vi "ep_Check Signaling Freuquency.vi"(8 "error in (no error)":errorcluster, 9 "nominal frequency value":dbl, 10 "phase voltage spectra":T2(array[cluster]), 11 "signaling frequency [Hz]":dbl) -> (0 "error out":errorcluster)   [LabVIEW 2014, in "NI_EP_Power Quality.lvlib"]
uses:
  <vilib>/addons/Electrical Power/PQ/NI_EP_Power Quality.lvlib
  <vilib>/addons/Electrical Power/PQ/Common/Controls/ep_AI Data Channel.ctl
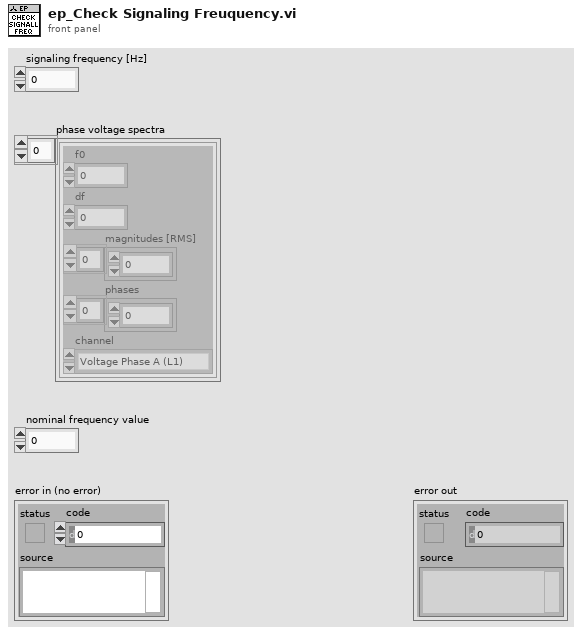
[diagram p1: front panel]
types:
  T1 = typedef "NI_EP_Power Quality.lvlib/ep_AI Data Channel.ctl" = enum16{"Voltage Phase A (L1)", "Voltage Phase B (L2)", "Voltage Phase C (L3)", "Voltage Phase N (Neutral)", "Current Phase A (L1)", "Current Phase B (L2)", "Current Phase C (L3)", "Current Phase N (Neutral)"}
  T2 = cluster{"f0":dbl, "df":dbl, "magnitudes [RMS]":dbl[], "phases":dbl[], "channel":T1}[]
  T3 = cluster{"f0":dbl, "df":dbl, "magnitudes [RMS]":dbl[], "phases":dbl[], "channel":T1}
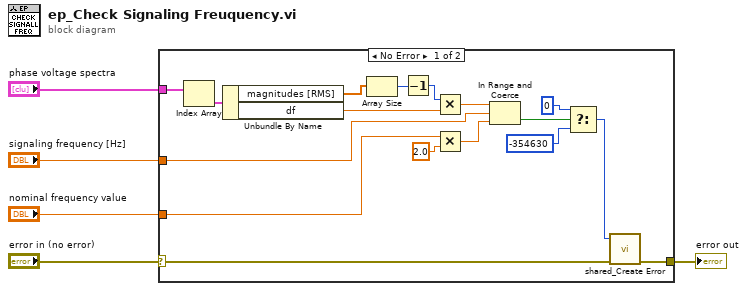
[diagram p0: block diagram]
diagram:
  n1 = case shown="No Error" "error in (no error)" {
    selector: "error in (no error)" -> [w7 w23]
    tunnel: "phase voltage spectra" -> [w20 _]
    tunnel: "signaling frequency [Hz]" -> [w16 _]
    tunnel: "nominal frequency value" -> [w13 _]
    tunnel: [w6 w23] -> w1
    frame No Error {
      n2 = Index Array(array=w20) -> (element=w19:T3)  [unwired: 1 in]
      n3 = Unbundle By Name(w19) -> ("magnitudes [RMS]"=w18:dbl[], "df"=w22:dbl)
      n4 = Array Size(array=w18) -> (size(s)=w17:i32)
      n5 = Decrement(x=w17) -> (x-1=w21:i32)
      n6 = Multiply(x=w21, y=w22) -> (x*y=w14:dbl)
      n7 = Multiply(x=w13, y=2.0) -> (x*y=w15:dbl)
      n8 = In Range and Coerce(upper limit=w14, x=w16, lower limit=w15) -> (In Range?=w9:bool)  [unwired: 1 out]
      n9 = Select(t=0 ("error code (0)"), s=w9, f=-354630 ("error code (0)")) -> (s? t:f=w8:i32)
      n10 = call <vilib>:"shared_Create Error.vi"("error in (no error)"=w7, "error code (0)"=w8) -> ("error out"=w6:errorcluster)  [unwired: 9 in]
    }
    frame Error {
    }
  }
  "error out" <- w1
